vi "ArmPathLength.vi"(4 "ArmPathIn":T1[](array[typedef])) -> (0 "Path Length":dbl, 1 "ArmPathOut":T1[](array[typedef]), 2 "IndexedPathLength":dbl[](array[numeric]))   [LabVIEW 2018]
uses:
  TypeDefs/ArmCoordinate.ctl
  ArgosLib/ArgosLib.lvlib
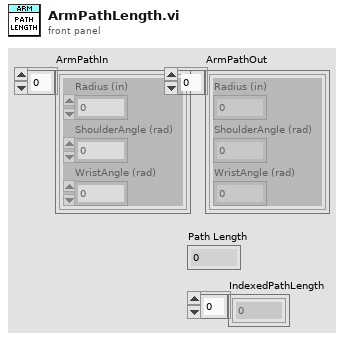
[diagram p1: front panel]
types:
  T1 = typedef "ArmCoordinate.ctl" = cluster{"Radius (in)":dbl, "ShoulderAngle (rad)":dbl, "WristAngle (rad)":dbl}
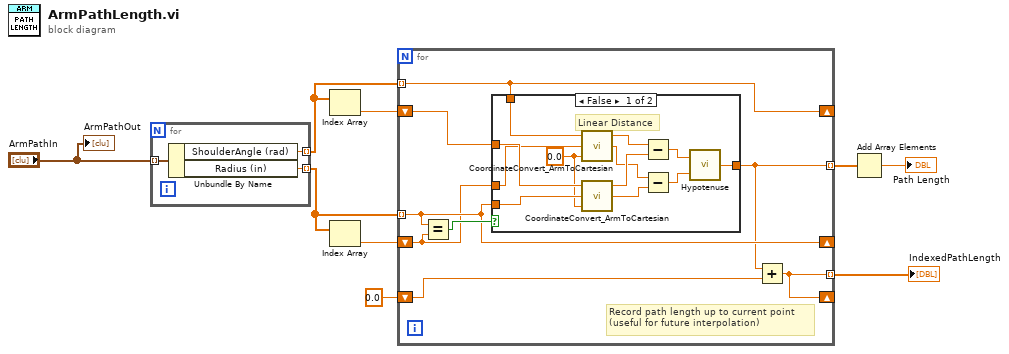
[diagram p0: block diagram]
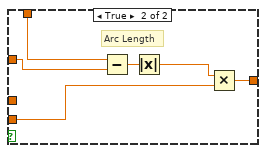
[diagram p2: hidden frame]
diagram:
  n1 = for {
    tunnel: "ArmPathIn" -> [w12] mode=indexing
    tunnel: [w11] -> w3 mode=indexing
    tunnel: [w10] -> w2 mode=indexing
    n2 = Unbundle By Name(w12) -> ("ShoulderAngle (rad)"=w11:dbl, "Radius (in)"=w10:dbl)
  }
  n3 = Index Array(array=w3) -> (element=w8:dbl)  [unwired: 1 in]
  n4 = Index Array(array=w2) -> (element=w7:dbl)  [unwired: 1 in]
  n5 = for {
    tunnel: w3 -> [w19] mode=indexing
    tunnel: w2 -> [w17] mode=indexing
    shift-right: [w17] -> _
    shift-left: w7 -> [w16]
    shift-right: [w19] -> _
    shift-left: w8 -> [w18]
    tunnel: [w14] -> w6 mode=indexing
    shift-right: [w15] -> _
    shift-left: 0.0 -> [w13]
    tunnel: [w15] -> w4 mode=indexing
    # "Record path length up to current point\n(useful for future interpolation)"
    n6 = Equal?(x=w17, y=w16) -> (x = y?=w20:bool)
    n7 = case shown="False" w20 {
      tunnel: w19 -> [w25 w36]
      tunnel: w16 -> [w23 _]
      tunnel: w17 -> [w22 w33]
      tunnel: [w26 w37] -> w14
      tunnel: w18 -> [w24 w35]
      frame False {
        w21 = 0.0 ("Wrist Angle (rad)")
        # "Linear Distance"
        n8 = call "CoordinateConvert_ArmToCartesian.vi"("Wrist Angle (rad)"=w21, "Radius (in)"=w23, "Shoulder Angle (rad)"=w25) -> ("Y (in)"=w30:dbl, "X (in)"=w32:dbl)  [unwired: 1 out]
        n9 = call "CoordinateConvert_ArmToCartesian.vi"("Wrist Angle (rad)"=w21, "Radius (in)"=w22, "Shoulder Angle (rad)"=w24) -> ("Y (in)"=w29:dbl, "X (in)"=w31:dbl)  [unwired: 1 out]
        n10 = Subtract(x=w32, y=w31) -> (x-y=w28:dbl)
        n11 = Subtract(x=w30, y=w29) -> (x-y=w27:dbl)
        n12 = call "Hypotenuse.vi"("Y"=w27, "X"=w28) -> ("Hypotenuse"=w26:dbl)
      }
      frame True {
        # "Arc Length"
        n13 = Subtract(x=w36, y=w35) -> (x-y=w38:dbl)
        n14 = Absolute Value(x=w38) -> (abs(x)=w34:dbl)
        n15 = Multiply(x=w34, y=w33) -> (x*y=w37:dbl)
      }
    }
    n16 = Add(x=w14, y=w13) -> (x+y=w15:dbl)
  }
  "IndexedPathLength" <- w4
  n17 = Add Array Elements(numeric array=w6) -> (sum=→"Path Length":dbl)
  "ArmPathOut" <- "ArmPathIn"
